vi "Initialize Debugging.vi"(4 "Error In":errorcluster) -> (0 "Error Out":errorcluster)   [LabVIEW 2014, in "Debugging.lvlib"]
uses:
  Debugging.lvlib
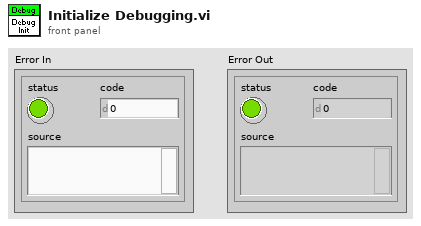
[diagram p1: front panel]
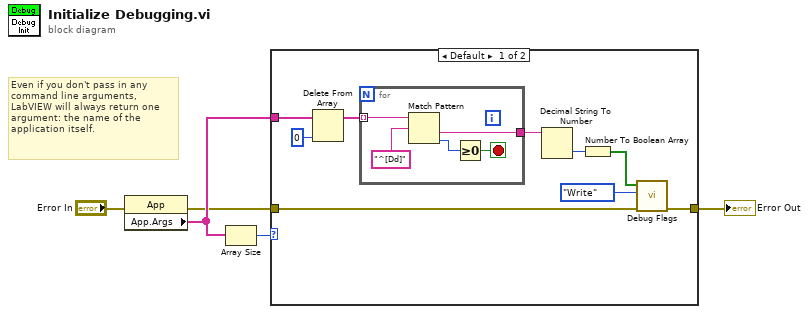
[diagram p0: block diagram]
diagram:
  # "Even if you don't pass in any command line arguments, LabVIEW will always return one argument: the name of the application itself."
  n1 = property class="App"(error in="Error In") -> (error out=w2:errorcluster, "App.Args"=w4:string[])  [unwired: 1 in, 1 out]
  n2 = Array Size(array=w4) -> (size(s)=w3:i32)
  n3 = case shown="Default" w3 {
    tunnel: w4 -> [w12 _]
    tunnel: w2 -> [w14 w20]
    tunnel: [w6 w20] -> w1
    frame Default {
      n4 = Delete From Array(array=w12, index=0) -> (array with subset deleted=w8:string[])  [unwired: 1 in, 1 out]
      n5 = for {
        tunnel: w8 -> [w19] mode=indexing
        tunnel: [w16] -> w11
        stop <- w17 stop-if-true
        n6 = Match Pattern(string=w19, regular expression="^[Dd]") -> (after substring=w16:string, offset past match=w18:i32)  [unwired: 1 in, 2 out]
        n7 = Greater Or Equal To 0?(x=w18) -> (x >= 0?=w17:bool)
      }
      n8 = Decimal String To Number(string=w11) -> (number=w10:i32)  [unwired: 2 in, 1 out]
      n9 = Number To Boolean Array(number=w10) -> (Boolean array=w9:bool[])
      n10 = call "Debug Flags.vi"("Error In"=w14, "Function"=enum16{"Read", "Write"}."Write", "Trace Flags In"=w9) -> ("Error Out"=w6:errorcluster)  [unwired: 3 in, 1 out]
    }
    frame 1 {
    }
  }
  "Error Out" <- w1
